vi "Dequeue Message.vi"(8 "error in (no error)":errorcluster, 9 "timeout in ms (-1)":i32, 11 "Queue in":refnum<class "Queue.lvclass">) -> (0 "error out":errorcluster, 1 "timed out?":bool, 2 "Message":refnum<class "Message.lvclass">, 3 "Queue out":refnum<class "Queue.lvclass">)   [LabVIEW 2019, in "Architecture.lvlib" / "Queue.lvclass"]
uses:
  Queue.lvclass
  Message/Message.lvclass
  Queue.lvclass/Queue.ctl
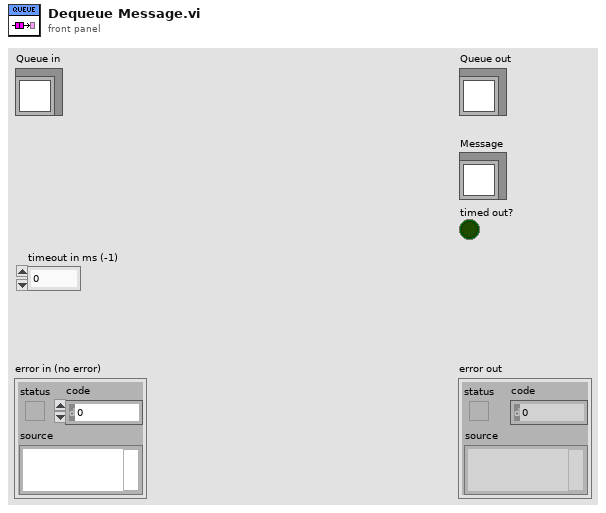
[diagram p1: front panel]
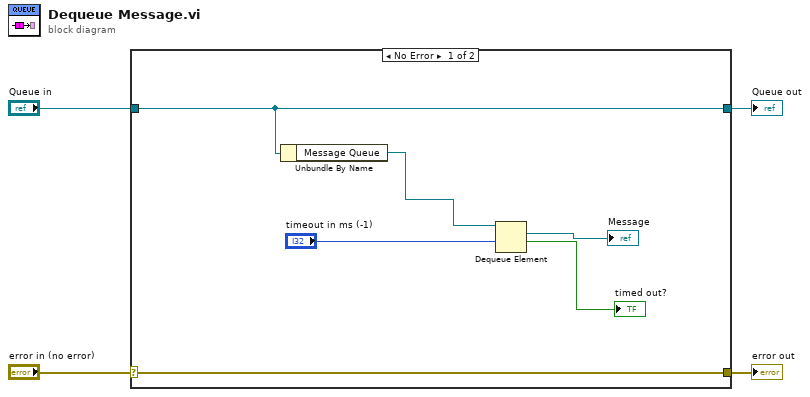
[diagram p0: block diagram]
diagram:
  n1 = case shown="No Error" "error in (no error)" {
    selector: "error in (no error)" -> [w10 w12]
    tunnel: [w10 w12] -> w3
    tunnel: [w9 w11] -> w1
    tunnel: "Queue in" -> [w9 w11]
    frame No Error {
      n2 = Unbundle By Name(w9) -> ("Message Queue"=w8:refnum<queue>)
      n3 = Dequeue Element(queue=w8, timeout in ms (-1)="timeout in ms (-1)") -> (element=→"Message":refnum<class "Message.lvclass">, timed out?=→"timed out?":bool)  [unwired: 1 in, 2 out]
    }
    frame Error {
    }
  }
  "error out" <- w3
  "Queue out" <- w1
